vi "LEDIntensityChangeWith_PWMsignal.vi"() -> ()   [LabVIEW 2022 SP3]
uses:
  <vilib>/DAQmx/write.llb/DAQmx Write (Digital Bool 1Line 1Point).vi
  <vilib>/DAQmx/create/channels.llb/DAQmx Create Channel (DO-Digital Output).vi
  <vilib>/DAQmx/miscellaneous.llb/DAQmx Fill In Error Info.vi
panel:
  in  "lines":tag
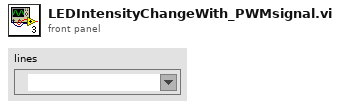
[diagram p1: front panel]
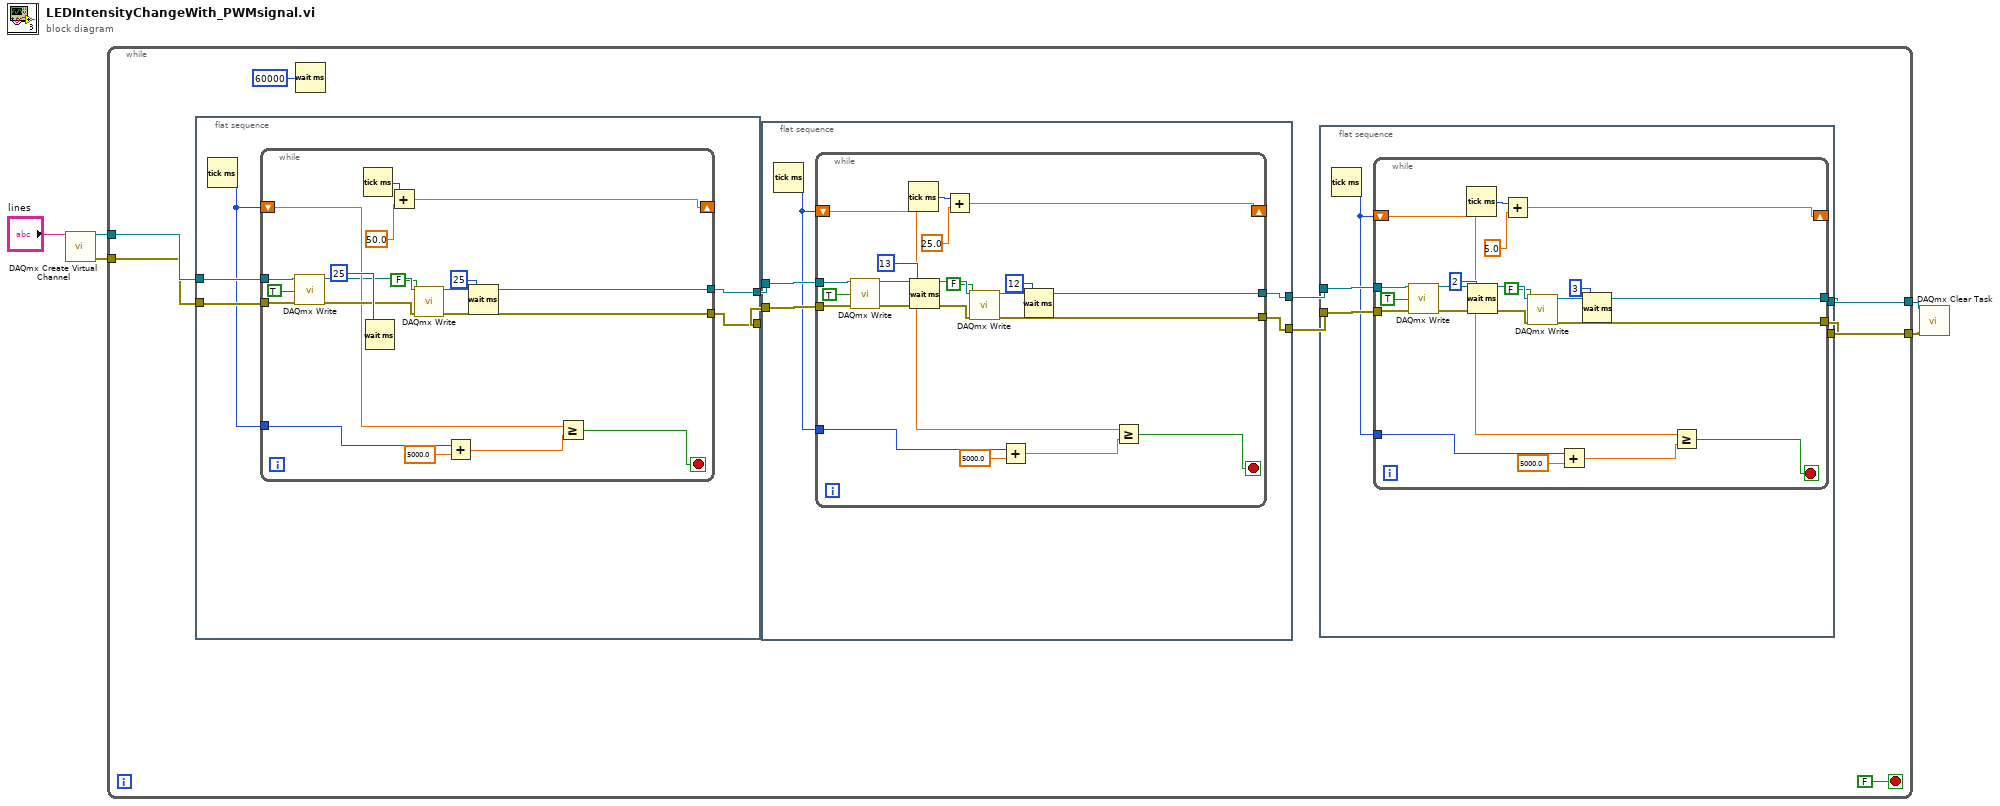
[diagram p0: block diagram]
diagram:
  n1 = call-poly <vilib>:"DAQmx Create Virtual Channel.vi"("lines"="lines") -> ("task out"=w5:refnum<k21>, "error out"=w4:errorcluster)  [unwired: 13 in]
  n2 = while {
    tunnel: w5 -> [w15]
    tunnel: w4 -> [w14]
    tunnel: [w9] -> w2
    tunnel: [w8] -> w1
    stop <- FALSE stop-if-true
    n3 = flat-sequence {
      tunnel: w15 -> [w66]
      tunnel: w14 -> [w65]
      tunnel: [w64] -> w13
      tunnel: [w63] -> w12
      frame #0 {
        n4 = Tick Count (ms)() -> (millisecond timer value=w62:u32)
        n5 = while {
          tunnel: w66 -> [w84]
          tunnel: w65 -> [w83]
          tunnel: [w78] -> w64
          tunnel: [w77] -> w63
          shift-right: [w74] -> _
          shift-left: w62 -> [w70]
          tunnel: w62 -> [w71]
          stop <- w73 stop-if-true
          n6 = call-poly <vilib>:"DAQmx Write.vi"("task/channels in"=w84, "data"=TRUE, "error in"=w83) -> ("task out"=w68:refnum<k21>, "error out"=w80:errorcluster)  [unwired: 10 in, 1 out]
          n7 = Tick Count (ms)() -> (millisecond timer value=w75:u32)
          n8 = Wait (ms)(milliseconds to wait=u32 25) -> ()  [unwired: 1 out]
          n9 = Add(x=w75, y=50.0) -> (x+y=w74:dbl)
          n10 = call-poly <vilib>:"DAQmx Write.vi"("task/channels in"=w68, "data"=FALSE, "error in"=w80) -> ("task out"=w78:refnum<k21>, "error out"=w77:errorcluster)  [unwired: 10 in, 1 out]
          n11 = Add(x=w71, y=5000.0) -> (x+y=w69:dbl)
          n12 = Wait (ms)(milliseconds to wait=u32 25) -> ()  [unwired: 1 out]
          n13 = Greater Or Equal?(x=w70, y=w69) -> (x >= y?=w73:bool)
        }
      }
    }
    n14 = Wait (ms)(milliseconds to wait=u32 60000) -> ()  [unwired: 1 out]
    n15 = flat-sequence {
      tunnel: w13 -> [w43]
      tunnel: w12 -> [w42]
      tunnel: [w41] -> w11
      tunnel: [w40] -> w10
      frame #0 {
        n16 = Tick Count (ms)() -> (millisecond timer value=w39:u32)
        n17 = while {
          tunnel: w43 -> [w61]
          tunnel: w42 -> [w60]
          tunnel: [w54] -> w41
          tunnel: [w53] -> w40
          shift-right: [w50] -> _
          shift-left: w39 -> [w46]
          tunnel: w39 -> [w47]
          stop <- w49 stop-if-true
          n18 = call-poly <vilib>:"DAQmx Write.vi"("task/channels in"=w61, "data"=TRUE, "error in"=w60) -> ("task out"=w57:refnum<k21>, "error out"=w56:errorcluster)  [unwired: 10 in, 1 out]
          n19 = Tick Count (ms)() -> (millisecond timer value=w51:u32)
          n20 = Wait (ms)(milliseconds to wait=u32 13) -> ()  [unwired: 1 out]
          n21 = Add(x=w51, y=25.0) -> (x+y=w50:dbl)
          n22 = call-poly <vilib>:"DAQmx Write.vi"("task/channels in"=w57, "data"=FALSE, "error in"=w56) -> ("task out"=w54:refnum<k21>, "error out"=w53:errorcluster)  [unwired: 10 in, 1 out]
          n23 = Add(x=w47, y=5000.0) -> (x+y=w45:dbl)
          n24 = Wait (ms)(milliseconds to wait=u32 12) -> ()  [unwired: 1 out]
          n25 = Greater Or Equal?(x=w46, y=w45) -> (x >= y?=w49:bool)
        }
      }
    }
    n26 = flat-sequence {
      tunnel: w11 -> [w20]
      tunnel: w10 -> [w19]
      tunnel: [w18] -> w9
      tunnel: [w17] -> w8
      frame #0 {
        n27 = Tick Count (ms)() -> (millisecond timer value=w16:u32)
        n28 = while {
          tunnel: w20 -> [w38]
          tunnel: w19 -> [w37]
          tunnel: [w31] -> w18
          tunnel: [w30] -> w17
          shift-right: [w27] -> _
          shift-left: w16 -> [w23]
          tunnel: w16 -> [w24]
          stop <- w26 stop-if-true
          n29 = call-poly <vilib>:"DAQmx Write.vi"("task/channels in"=w38, "data"=TRUE, "error in"=w37) -> ("task out"=w34:refnum<k21>, "error out"=w33:errorcluster)  [unwired: 10 in, 1 out]
          n30 = Tick Count (ms)() -> (millisecond timer value=w28:u32)
          n31 = Wait (ms)(milliseconds to wait=u32 2) -> ()  [unwired: 1 out]
          n32 = Add(x=w28, y=5.0) -> (x+y=w27:dbl)
          n33 = call-poly <vilib>:"DAQmx Write.vi"("task/channels in"=w34, "data"=FALSE, "error in"=w33) -> ("task out"=w31:refnum<k21>, "error out"=w30:errorcluster)  [unwired: 10 in, 1 out]
          n34 = Add(x=w24, y=5000.0) -> (x+y=w22:dbl)
          n35 = Wait (ms)(milliseconds to wait=u32 3) -> ()  [unwired: 1 out]
          n36 = Greater Or Equal?(x=w23, y=w22) -> (x >= y?=w26:bool)
        }
      }
    }
  }
  n37 = call <vilib>:"DAQmx Clear Task.vi"("task in"=w2, "error in"=w1) -> ()  [unwired: 13 in, 1 out]
